vi "Set_supply_with_boardhandle.vi"(6 "Current Limit (0.00 uA)":sgl format="%.2g", 7 "Channel (0)":u8, 8 "error in (no error)":errorcluster, 9 "Voltage Max (0.0 V)":u16 max=9999, 10 "Voltage Level (0.0 V)":dbl format="%.1g", 11 "BoardHandle":T1) -> (0 "error out":errorcluster, 3 "BoardHandle out":T1)   [LabVIEW 2018]
uses:
  <instrlib>/CAEN PSM/CAEN PSM.lvlib
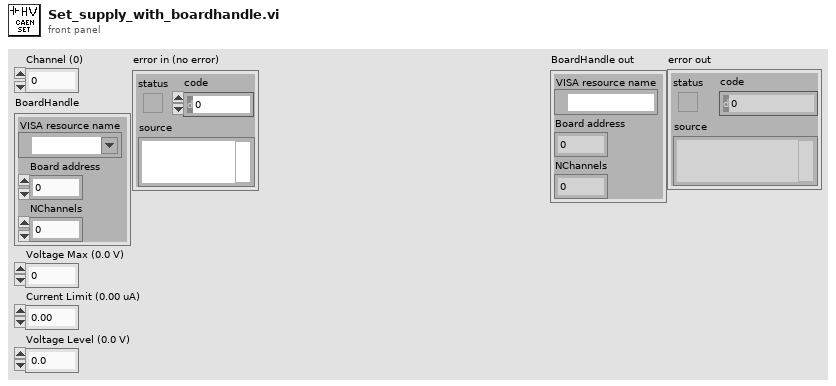
[diagram p1: front panel]
types:
  T1 = cluster{"VISA resource name":refnum<visa-resource-name>, "Board address":u8, "NChannels":u8}
  T2 = typedef "CAEN PSM.lvlib/BoardHandle.ctl" = cluster{"VISA resource name":refnum<visa-resource-name>, "Board address":u8, "NChannels":u8}
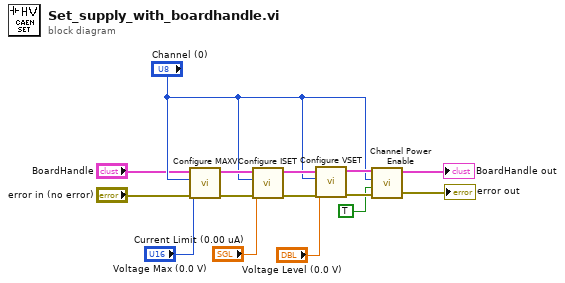
[diagram p0: block diagram]
diagram:
  n1 = call <instrlib>:"Configure MAXV.vi"("error in (no error)"="error in (no error)", "Voltage Max (0.0 V)"="Voltage Max (0.0 V)", "Channel (0)"="Channel (0)", "BoardHandle"="BoardHandle") -> ("error out"=w13:errorcluster, "BoardHandle out"=w15:T2)  [unwired: 6 in]
  n2 = call <instrlib>:"Configure ISET.vi"("error in (no error)"=w13, "Current Limit (0.00 uA)"="Current Limit (0.00 uA)", "Channel (0)"="Channel (0)", "BoardHandle"=w15) -> ("error out"=w12:errorcluster, "BoardHandle out"=w14:T2)  [unwired: 6 in]
  n3 = call <instrlib>:"Configure VSET.vi"("error in (no error)"=w12, "Voltage Level (0.0 V)"="Voltage Level (0.0 V)", "Channel (0)"="Channel (0)", "BoardHandle"=w14) -> ("error out"=w11:errorcluster, "BoardHandle out"=w10:T2)  [unwired: 6 in]
  n4 = call <instrlib>:"Channel Power Enable.vi"("error in (no error)"=w11, "Enable (OFF)"=TRUE, "Channel (0)"="Channel (0)", "BoardHandle"=w10) -> ("error out"=→"error out":errorcluster, "BoardHandle out"=→"BoardHandle out":T2)  [unwired: 6 in]
